vi "test-VAttributes-Merge.vi"(8 "error in (no error)":errorcluster, 11 "TestCase in":refnum<class "MyTestCase.lvclass">) -> (0 "error out":errorcluster, 3 "TestCase out":refnum<class "MyTestCase.lvclass">)   [LabVIEW 2019, in "MyTestCase.lvclass"]
uses:
  MyTestCase.lvclass
  <vilib>/addons/_JKI Toolkits/VI Tester/TestCase.llb/TestCase.lvclass
  lv-apt-json-file.lvlib
  C:/Program Files (x86)/National Instruments/LabVIEW 2019/vi.lib/addons/_JKI Toolkits/VI Tester/TestCase.llb/TestCase.lvclass
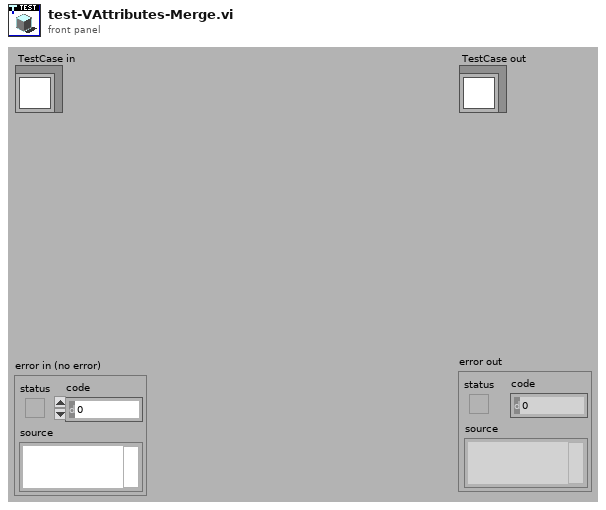
[diagram p1: front panel]
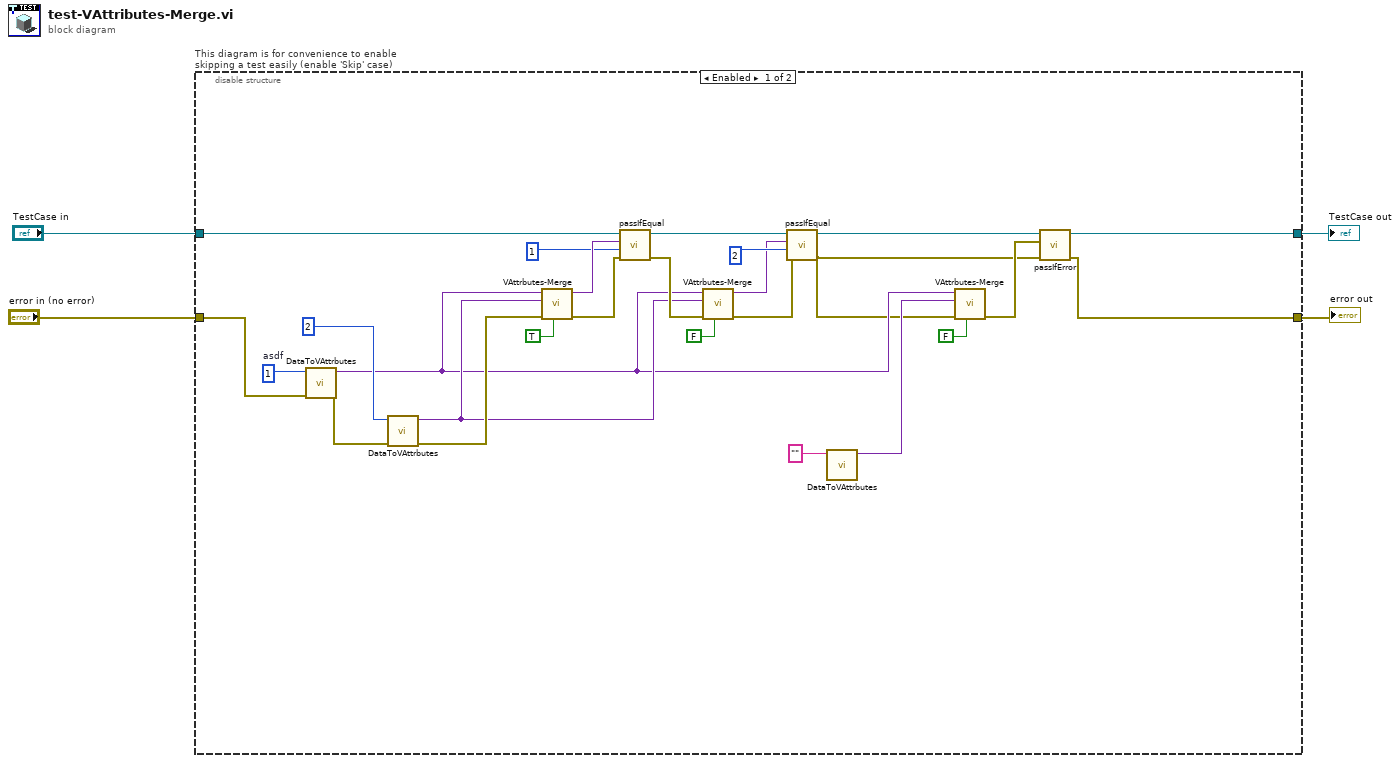
[diagram p0: block diagram]
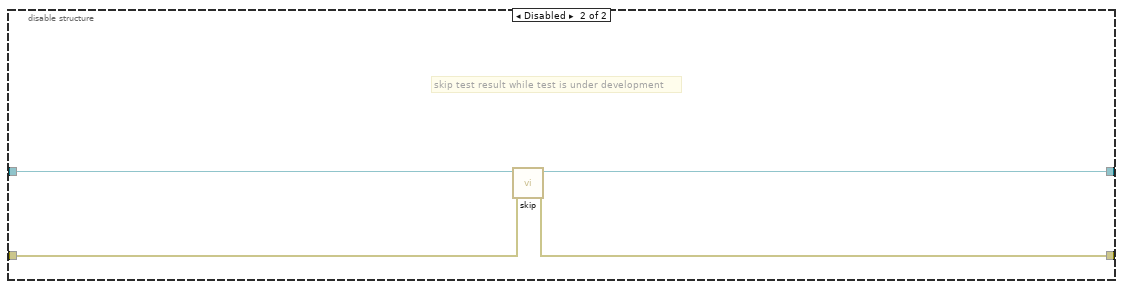
[diagram p2: hidden frame]
diagram:
  n1 = disable-structure "This diagram is for convenience to enable skipping a test easily (enable 'Skip' case)" shown="Enabled" {
    disable-tunnel: "TestCase in" -> [w25 w34]
    disable-tunnel: [w12 w32] -> w1
    disable-tunnel: [w5 w33] -> w3
    disable-tunnel: "error in (no error)" -> [w26 w31]
    frame Enabled {
      w30 = 1  # asdf
      n2 = call "DataToVAttrbutes.vi"("error in (no error)"=w26, "data"=w30) -> ("error out"=w28:errorcluster, "VAttributes"=w9:variant)  [unwired: 8 in]
      n3 = call "DataToVAttrbutes.vi"("error in (no error)"=w28, "data"=2) -> ("error out"=w27:errorcluster, "VAttributes"=w15:variant)  [unwired: 8 in]
      n4 = call "VAttrbutes-Merge.vi"("If exist? Skip(T)/Overwrite(F)"=TRUE, "error in (no error)"=w27, "VAttributes B"=w15, "VAttributes A"=w9) -> ("error out"=w19:errorcluster, "VAttributes A after B->A"=w24:variant)  [unwired: 6 in]
      n5 = call-dynamic "passIfEqual.vi"("error in (no error)"=w19, "y"=1, "x"=w24, "TestCase in"=w25) -> ("error out"=w18:errorcluster, "TestCase out"=w16:refnum<class "MyTestCase.lvclass">)  [unwired: 6 in]
      n6 = call "VAttrbutes-Merge.vi"("If exist? Skip(T)/Overwrite(F)"=FALSE, "error in (no error)"=w18, "VAttributes B"=w15, "VAttributes A"=w9) -> ("error out"=w17:errorcluster, "VAttributes A after B->A"=w13:variant)  [unwired: 6 in]
      n7 = call-dynamic "passIfEqual.vi"("error in (no error)"=w17, "y"=2, "x"=w13, "TestCase in"=w16) -> ("error out"=w6:errorcluster, "TestCase out"=w14:refnum<class "MyTestCase.lvclass">)  [unwired: 6 in]
      n8 = call "DataToVAttrbutes.vi"("data"="") -> ("VAttributes"=w8:variant)  [unwired: 9 in, 1 out]
      n9 = call "VAttrbutes-Merge.vi"("If exist? Skip(T)/Overwrite(F)"=FALSE, "error in (no error)"=w6, "VAttributes B"=w8, "VAttributes A"=w9) -> ("error out"=w7:errorcluster)  [unwired: 6 in, 1 out]
      n10 = call-dynamic "passIfError.vi"("error in (no error)"=w6, "error"=w7, "TestCase in"=w14) -> ("error out"=w5:errorcluster, "TestCase out"=w12:refnum<class "MyTestCase.lvclass">)  [unwired: 7 in]
    }
    frame Disabled {
      # "skip test result while test is under development"
      n11 = call <vilib>:"skip.vi"("error in (no error)"=w31, "TestCase in"=w34) -> ("error out"=w33:errorcluster, "TestCase out"=w32:refnum<class "MyTestCase.lvclass">)  [unwired: 8 in]
    }
  }
  "error out" <- w3
  "TestCase out" <- w1
